vi "str to double.vi"(2 "String":string) -> (6 "double":dbl)   [LabVIEW 2013]
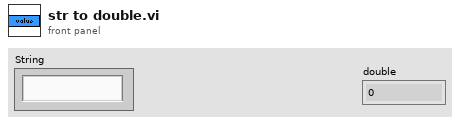
[diagram p1: front panel]
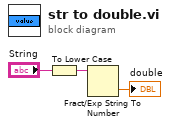
[diagram p0: block diagram]
diagram:
  n1 = To Lower Case(string="String") -> (all lower case string=w2:string)
  n2 = Fract/Exp String To Number(string=w2) -> (number=→"double":dbl)  [unwired: 3 in, 1 out]
